vi "EnQueue Trigger.vi"(0 "Queue in":refnum<queue>, 5 "System Triggers":T1, 7 "Trigger Data":variant, 9 "Timeout (0)":i32, 11 "error in (no error)":errorcluster) -> (4 "Queue out":refnum<queue>, 15 "error out":errorcluster)   [LabVIEW 2015, in "TLB` Template.lvlib"]
doc: "TLB Prime - Application Template 1.3.0.24\nNorm Kirchner, NI Systems Engineering - NI\nCopyright (c) 2014, NI"
uses:
  TLB` Template.lvlib
  System Trigger.ctl
  System Trigger Element.ctl
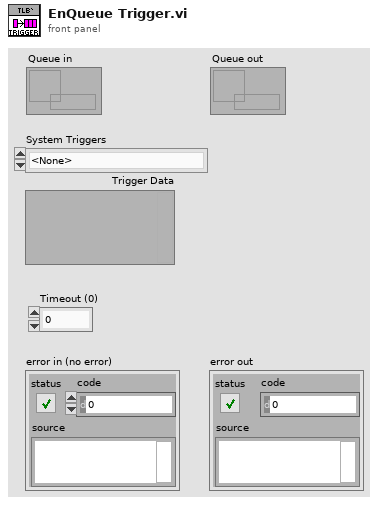
[diagram p1: front panel]
types:
  T1 = typedef "TLB` Template.lvlib/System Trigger.ctl" = enum16{"<None>", "Cache User Parameters", "Close Application"}
  T2 = typedef "TLB` Template.lvlib/System Trigger Element.ctl" = cluster{"System Triggers":T1, "Trigger Data":variant}
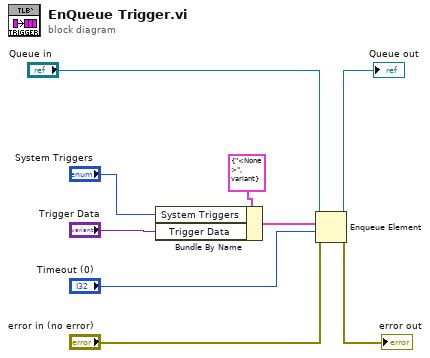
[diagram p0: block diagram]
diagram:
  n1 = Bundle By Name(cluster=T2 {"System Triggers"=enum."<None>", "Trigger Data"=variant} ("element"), "System Triggers"="System Triggers", "Trigger Data"="Trigger Data") -> (w7:T2)
  n2 = Enqueue Element(queue="Queue in", element=w7, timeout in ms (-1)="Timeout (0)", error in (no error)="error in (no error)") -> (queue out=→"Queue out":refnum<queue>, error out=→"error out":errorcluster)  [unwired: 1 out]
